vi "Run Auto Score.vi"(11 "Zip":path) -> (3 "Result":T1 {"Score" format="%#.6f"})   [LabVIEW 2024, in "Wordle Scorer.lvlib"]
uses:
  Wordle Scorer.lvlib
  Scoring Result.ctl
  <vilib>/Utility/error.llb/DialogType.ctl
  Result.ctl
  <vilib>/IlluminatedG/IG Inspector/Inspector/SoL Inspector.lvlib
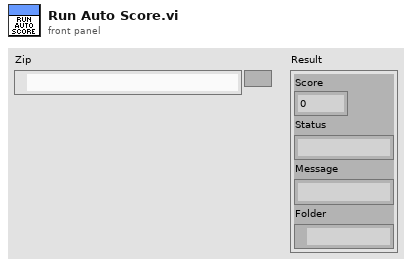
[diagram p1: front panel]
types:
  T1 = typedef "Wordle Scorer.lvlib/Scoring Result.ctl" = cluster{"Score":dbl, "Status":string, "Message":string, "Folder":path}
  T2 = typedef "DialogType.ctl" = u16
  T3 = typedef "SoL Inspector.lvlib/Inspector Config.ctl" = cluster{"Inspections (All)":T4[], "Disallowed ClassNames":string[], "Disallowed Functions":string[], "Disallowed SubVI Paths":string[], "Allowed Properties":string[], "Allowed Invoke Nodes":string[]}
  T4 = typedef "SoL Inspector.lvlib/Inspection.ctl" = enum16{"ClassName", "Functions", "CallLibrary", "SubVIs", "FileIO", "Invoke Nodes", "Properties", "Growable Functions"}
  T5 = typedef "Wordle Scorer.lvlib/Result.ctl" = enum16{"failed", "complete", "error", "timeout", "ineligible"}
  T6 = typedef "Wordle Scorer.lvlib/Solver VI Ref Type.ctl" = refnum<vi>
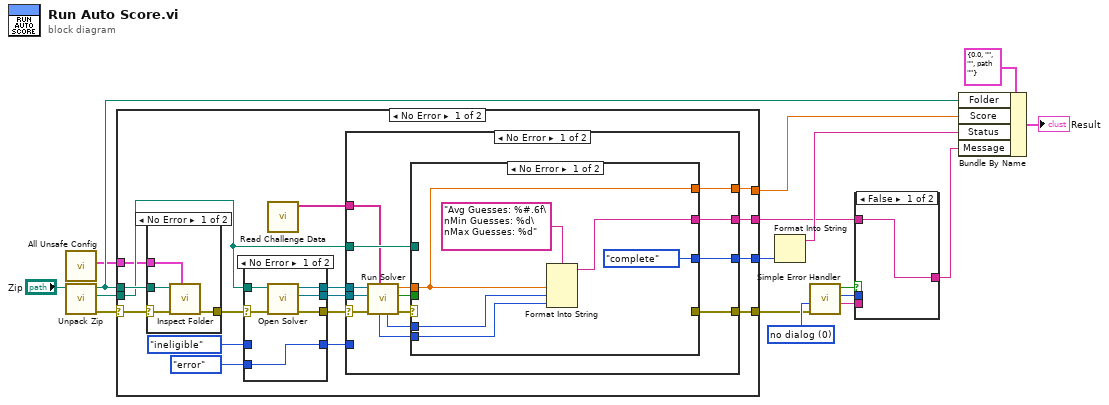
[diagram p0: block diagram]
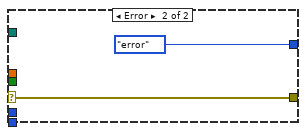
[diagram p2: hidden frame]
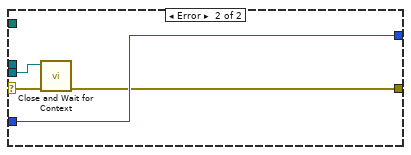
[diagram p3: hidden frame]
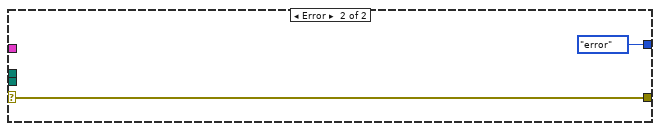
[diagram p6: hidden frame]
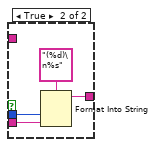
[diagram p7: hidden frame]
diagram:
  w9 = T2 0 items=["no dialog", "OK message", "continue or stop message", "OK message + warnings", "continue/stop + warnings"] ("type of dialog (OK msg:1)")
  n1 = call <vilib>:"All Unsafe Config.vi"() -> ("All Unsafe Config"=w1:T3)  [unwired: 11 in]
  n2 = call "Unpack Zip.vi"("Zip"="Zip") -> ("error out"=w16:errorcluster, "Solver VI"=w13:path, "Folder"=w5:path)  [unwired: 8 in]
  n3 = case shown="No Error" w16 {
    selector: w16 -> [w33 w73]
    tunnel: w5 -> [w29 _]
    tunnel: w13 -> [w22 _]
    tunnel: [w25 Result."error" ("Result")] -> w8
    tunnel: [w24 w73] -> w7
    tunnel: [w23 _] -> w6
    tunnel: [w21 _] -> w2
    tunnel: w1 -> [w20 _]
    frame No Error {
      n4 = case shown="No Error" w33 {
        selector: w33 -> [w71 w72]
        tunnel: w29 -> [w69 _]
        tunnel: [w70 w72] -> w32
        tunnel: w20 -> [w68 _]
        frame No Error {
          n5 = call <vilib>:"Inspect Folder.vi"("Inspector Config"=w68, "error in (no error)"=w71, "Folder"=w69) -> ("error out"=w70:errorcluster)  [unwired: 6 in, 2 out]
        }
        frame Error {
        }
      }
      n6 = case shown="No Error" w32 {
        selector: w32 -> [w64 w67]
        tunnel: w22 -> [w65 _]
        tunnel: [w63 _] -> w30
        tunnel: [w62 w67] -> w31
        tunnel: [w61 w66] -> w27
        tunnel: Result."error" ("Result") -> [w61 _]
        tunnel: Result."ineligible" ("Result") -> [_ w66]
        tunnel: [w60 _] -> w19
        frame No Error {
          n7 = call "Open Solver.vi"("error in (no error)"=w64, "Solver Path"=w65) -> ("error IO"=w62:errorcluster, "Scorer Context"=w60:refnum<vi>, "Solver VI"=w63:T6)  [unwired: 7 in]
        }
        frame Error {
        }
      }
      n8 = call "Read Challenge Data.vi"() -> ("Word List"=w18:string[])  [unwired: 10 in, 1 out]
      n9 = case shown="No Error" w31 {
        selector: w31 -> [w34 w59]
        tunnel: w30 -> [w39 _]
        tunnel: [w43 w57] -> w24
        tunnel: w22 -> [w44 _]
        tunnel: [w42 _] -> w23
        tunnel: [w41 w58] -> w25
        tunnel: w27 -> [_ w58]
        tunnel: [w40 _] -> w21
        tunnel: w19 -> [w38 w56]
        tunnel: w18 -> [w37 _]
        frame No Error {
          n10 = call "Run Solver.vi"("Words"=w37, "error in"=w34, "Scorer Context"=w38, "Solver Ref"=w39) -> ("error out"=w47:errorcluster, "Success"=w46:bool, "Avg Guesses"=w45:dbl, "Min Guesses"=w36:i32, "Max Guesses"=w35:i32)  [unwired: 3 in]
          n11 = case shown="No Error" w47 {
            selector: w47 -> [_ w55]
            tunnel: w46 -> [_ _]
            tunnel: w45 -> [w52 _]
            tunnel: w44 -> [_ _]
            tunnel: [_ w55] -> w43
            tunnel: [w52 _] -> w42
            tunnel: [Result."complete" ("Result") Result."error" ("Result")] -> w41
            tunnel: [w49 _] -> w40
            tunnel: w36 -> [w51 _]
            tunnel: w35 -> [w50 _]
            frame No Error {
              n12 = Format Into String(format string="Avg Guesses: %#.6f\nMin Guesses: %d\nMax Guesses: %d", w52, w51, w50) -> (resulting string=w49:string)  [unwired: 2 in, 1 out]
            }
            frame Error {
            }
          }
        }
        frame Error {
          n13 = call "Close and Wait for Context.vi"("error in (no error)"=w59, "Scorer Context"=w56) -> ("error out"=w57:errorcluster)  [unwired: 9 in]
        }
      }
    }
    frame Error {
    }
  }
  n14 = Format Into String(w8) -> (resulting string=w4:string)  [unwired: 3 in, 1 out]
  n15 = call <vilib>:"Simple Error Handler.vi"("type of dialog (OK msg:1)"=w9, "error in (no error)"=w7) -> ("error?"=w12:bool, "code out"=w11:i32, "source out"=w10:string)  [unwired: 3 in, 2 out]
  n16 = case shown="False" w12 {
    tunnel: w10 -> [_ w77]
    tunnel: w11 -> [_ w78]
    tunnel: w2 -> [w75 _]
    tunnel: [w75 w76] -> w3
    frame False {
    }
    frame True {
      n17 = Format Into String(format string="(%d)\n%s", w78, w77) -> (resulting string=w76:string)  [unwired: 2 in, 1 out]
    }
  }
  n18 = Bundle By Name(cluster=T1 {"Score"=0.0, "Status"="", "Message"="", "Folder"=path ""} ("Scoring Result"), "Folder"=w5, "Score"=w6, "Status"=w4, "Message"=w3) -> (→"Result":T1)
